vi "TextLog-Flush Log.vi"(0 "State in":T1) -> (4 "State out":T1)   [LabVIEW 2020]
uses:
  TextLog-State.ctl
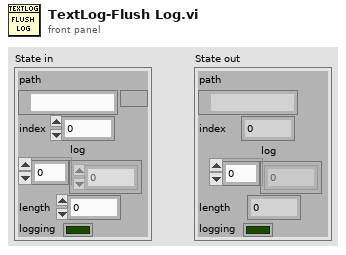
[diagram p1: front panel]
types:
  T1 = typedef "TextLog-State.ctl" = cluster{"path":path, "index":i32, "log":u8[], "length":i32, "logging":bool}
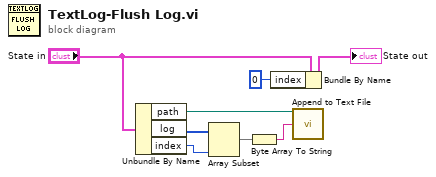
[diagram p0: block diagram]
diagram:
  n1 = Unbundle By Name("State in") -> ("path"=w6:path, "log"=w5:u8[], "index"=w4:i32)
  n2 = Array Subset(array=w5, length=w4) -> (w3:u8[])  [unwired: 1 in]
  n3 = Byte Array To String(unsigned byte array=w3) -> (string=w2:string)
  n4 = Bundle By Name(cluster="State in", "index"=0) -> (→"State out":T1)
  n5 = call "Append to Text File.vi"("file path"=w6, "text"=w2) -> ()  [unwired: 12 in, 2 out]
